vi "Get Control Data Type.vi"(8 "error in (no error)":errorcluster, 11 "Ctl Refnum":refnum<vi>) -> (0 "error out":errorcluster, 3 "Type":refnum<class "LVType.lvclass">)   [LabVIEW 2020, in "LVDataTypes.lvlib"]
uses:
  <vilib>/AppBuilder/Engine/WebServiceDescription/LVDataTypes/LVDataTypes.lvlib
  <vilib>/AppBuilder/Engine/WebServiceDescription/LVDataTypes/LVType/LVType.lvclass
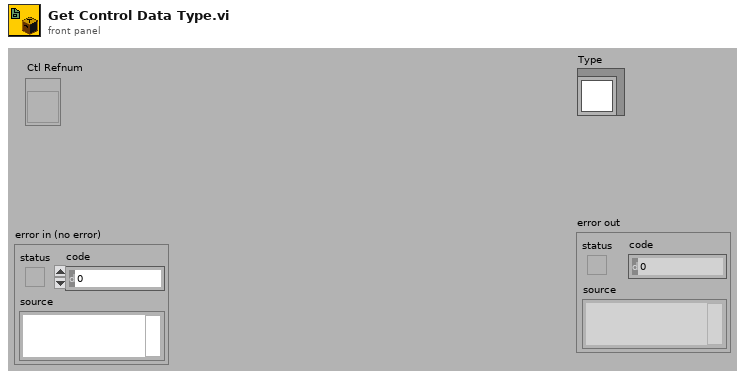
[diagram p1: front panel]
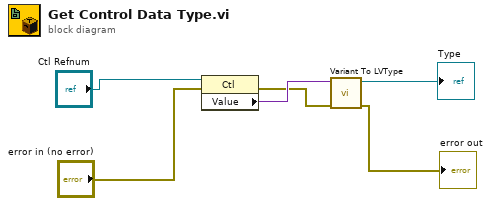
[diagram p0: block diagram]
diagram:
  n1 = property on="Property Node" class="Ctl"(reference="Ctl Refnum", error in="error in (no error)") -> (error out=w3:errorcluster, "Value"=w4:variant)  [unwired: 1 out]
  n2 = call <vilib>:"Variant To LVType.vi"("error in (no error)"=w3, "Variant"=w4) -> ("error out"=→"error out":errorcluster, "LVType"=→"Type":refnum<class "LVType.lvclass">)  [unwired: 8 out]
